vi "Close Command.vi"(0 "SLSC Local in":refnum<class "SLSC Local.lvclass">, 5 "command":refnum<k21>, 11 "error in (no error)":errorcluster) -> (4 "SLSC Local out":refnum<class "SLSC Local.lvclass">, 15 "error out":errorcluster)   [LabVIEW 2015, in "SLSC Local.lvclass"]
uses:
  SLSC Local.lvclass
  <vilib>/SLSC/SLSC.lvlib
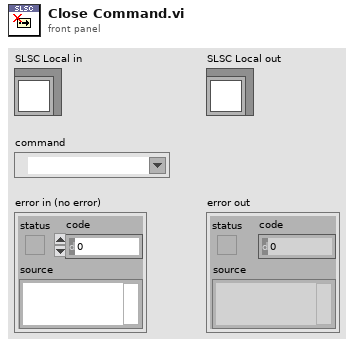
[diagram p1: front panel]
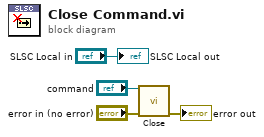
[diagram p0: block diagram]
diagram:
  n1 = call-poly <vilib>:"Close.vi"("command"="command", "error in (no error)"="error in (no error)") -> ("error out"=→"error out":errorcluster)  [unwired: 13 in]
  "SLSC Local out" <- "SLSC Local in"
